vi "Write Connection Ref.vi"(8 "error in (no error)":errorcluster, 10 "Connection Ref":variant, 11 "PXIe 2737 in":refnum<class "PXIe 2737.lvclass">) -> (0 "error out":errorcluster, 3 "PXIe 2737 out":refnum<class "PXIe 2737.lvclass">)   [LabVIEW 2021, in "S-Matrix.lvlib" / "PXIe 2737.lvclass"]
uses:
  PXIe 2737.lvclass
  PXIe 2737.lvclass/PXIe 2737.ctl
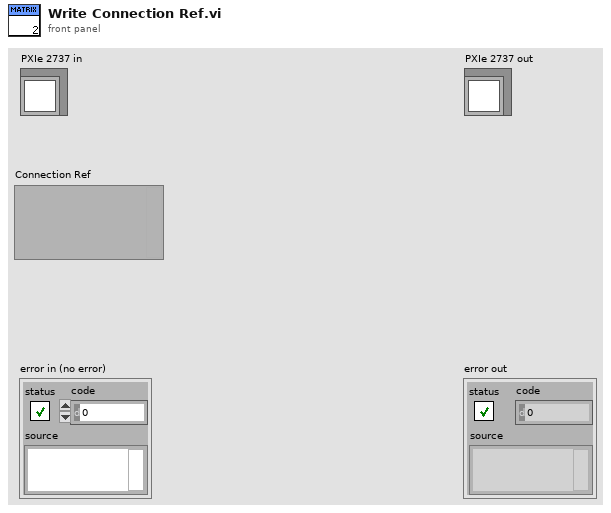
[diagram p1: front panel]
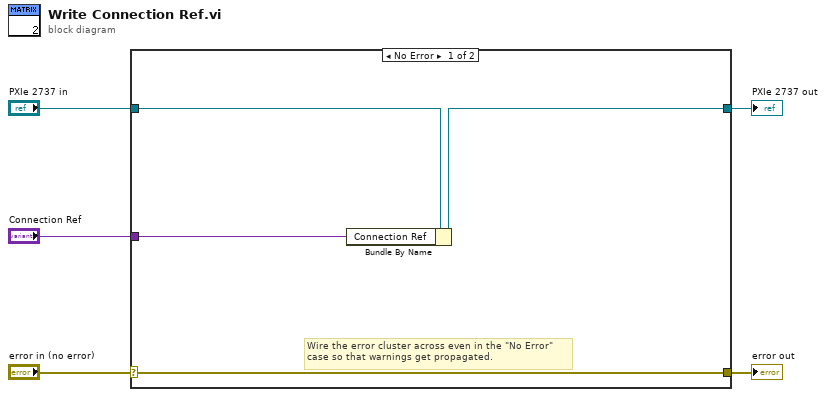
[diagram p0: block diagram]
diagram:
  n1 = case shown="No Error" "error in (no error)" {
    selector: "error in (no error)" -> [w8 w11]
    tunnel: [w8 w11] -> w4
    tunnel: [w7 w10] -> w2
    tunnel: "PXIe 2737 in" -> [w9 w10]
    tunnel: "Connection Ref" -> [w6 _]
    frame No Error {
      # "Wire the error cluster across even in the \"No Error\"\ncase so that warnings get propagated."
      n2 = Bundle By Name(cluster=w9, "Connection Ref"=w6) -> (w7:refnum<class "PXIe 2737.lvclass">)
    }
    frame Error {
    }
  }
  "error out" <- w4
  "PXIe 2737 out" <- w2
